vi "App - analyze RUS V6.vi"() -> ()   [LabVIEW 2021] (continued)
{"temperature"=59.124, "temperature str"="59.12400", "file path"=path "D:/Data/Ultrasound/LSCO/LSCO22__130814c/5_Cooling_2nd_try/September_2014/091714/59.12400K_500_2500_2.10000V_0.00000T_Sep17-2014__08-44-26_001_091714.bin", "last mod"=timestamp(3493802666 s since 1904-01-01), "file name str"="D:\\Data\\Ultrasound\\LSCO\\LSCO22__130814c\\5_Cooling_2nd_try\\September_2014\\091714\\59.12400K_500_2500_2.10000V_0.00000T_Sep17-2014__08-44-26_001_091714.bin", "mod time(min)"=58230044.43333333, "file format"=enum."binary", "power(V)"=2.1, "Magn Field(T) "=0.0}, {"temperature"=59.067, "temperature str"="59.06700", "file path"=path "D:/Data/Ultrasound/LSCO/LSCO22__130814c/5_Cooling_2nd_try/September_2014/091714/59.06700K_500_2500_2.10000V_0.00000T_Sep17-2014__08-45-45_001_091714.bin", "last mod"=timestamp(3493802745 s since 1904-01-01), "file name str"="D:\\Data\\Ultrasound\\LSCO\\LSCO22__130814c\\5_Cooling_2nd_try\\September_2014\\091714\\59.06700K_500_2500_2.10000V_0.00000T_Sep17-2014__08-45-45_001_091714.bin", "mod time(min)"=58230045.75, "file format"=enum."binary", "power(V)"=2.1, "Magn Field(T) "=0.0}, {"temperature"=59.005, "temperature str"="59.00500", "file path"=path "D:/Data/Ultrasound/LSCO/LSCO22__130814c/5_Cooling_2nd_try/September_2014/091714/59.00500K_500_2500_2.10000V_0.00000T_Sep17-2014__08-47-05_001_091714.bin", "last mod"=timestamp(3493802825 s since 1904-01-01), "file name str"="D:\\Data\\Ultrasound\\LSCO\\LSCO22__130814c\\5_Cooling_2nd_try\\September_2014\\091714\\59.00500K_500_2500_2.10000V_0.00000T_Sep17-2014__08-47-05_001_091714.bin", "mod time(min)"=58230047.083333336, "file format"=enum."binary", "power(V)"=2.1, "Magn Field(T) "=0.0}, {"temperature"=58.947, "temperature str"="58.94700", "file path"=path "D:/Data/Ultrasound/LSCO/LSCO22__130814c/5_Cooling_2nd_try/September_2014/091714/58.94700K_500_2500_2.10000V_0.00000T_Sep17-2014__08-48-24_001_091714.bin", "last mod"=timestamp(3493802904 s since 1904-01-01), "file name str"="D:\\Data\\Ultrasound\\LSCO\\LSCO22__130814c\\5_Cooling_2nd_try\\September_2014\\091714\\58.94700K_500_2500_2.10000V_0.00000T_Sep17-2014__08-48-24_001_091714.bin", "mod time(min)"=58230048.4, "file format"=enum."binary", "power(V)"=2.1, "Magn Field(T) "=0.0}, {"temperature"=58.886, "temperature str"="58.88600", "file path"=path "D:/Data/Ultrasound/LSCO/LSCO22__130814c/5_Cooling_2nd_try/September_2014/091714/58.88600K_500_2500_2.10000V_0.00000T_Sep17-2014__08-49-43_001_091714.bin", "last mod"=timestamp(3493802983 s since 1904-01-01), "file name str"="D:\\Data\\Ultrasound\\LSCO\\LSCO22__130814c\\5_Cooling_2nd_try\\September_2014\\091714\\58.88600K_500_2500_2.10000V_0.00000T_Sep17-2014__08-49-43_001_091714.bin", "mod time(min)"=58230049.71666667, "file format"=enum."binary", "power(V)"=2.1, "Magn Field(T) "=0.0}, {"temperature"=58.831, "temperature str"="58.83100", "file path"=path "D:/Data/Ultrasound/LSCO/LSCO22__130814c/5_Cooling_2nd_try/September_2014/091714/58.83100K_500_2500_2.10000V_0.00000T_Sep17-2014__08-51-03_001_091714.bin", "last mod"=timestamp(3493803063 s since 1904-01-01), "file name str"="D:\\Data\\Ultrasound\\LSCO\\LSCO22__130814c\\5_Cooling_2nd_try\\September_2014\\091714\\58.83100K_500_2500_2.10000V_0.00000T_Sep17-2014__08-51-03_001_091714.bin", "mod time(min)"=58230051.05, "file format"=enum."binary", "power(V)"=2.1, "Magn Field(T) "=0.0}, {"temperature"=58.769, "temperature str"="58.76900", "file path"=path "D:/Data/Ultrasound/LSCO/LSCO22__130814c/5_Cooling_2nd_try/September_2014/091714/58.76900K_500_2500_2.10000V_0.00000T_Sep17-2014__08-52-22_001_091714.bin", "last mod"=timestamp(3493803142 s since 1904-01-01), "file name str"="D:\\Data\\Ultrasound\\LSCO\\LSCO22__130814c\\5_Cooling_2nd_try\\September_2014\\091714\\58.76900K_500_2500_2.10000V_0.00000T_Sep17-2014__08-52-22_001_091714.bin", "mod time(min)"=58230052.36666667, "file format"=enum."binary", "power(V)"=2.1, "Magn Field(T) "=0.0}, {"temperature"=58.708, "temperature str"="58.70800", "file path"=path "D:/Data/Ultrasound/LSCO/LSCO22__130814c/5_Cooling_2nd_try/September_2014/091714/58.70800K_500_2500_2.10000V_0.00000T_Sep17-2014__08-53-41_001_091714.bin", "last mod"=timestamp(3493803221 s since 1904-01-01), "file name str"="D:\\Data\\Ultrasound\\LSCO\\LSCO22__130814c\\5_Cooling_2nd_try\\September_2014\\091714\\58.70800K_500_2500_2.10000V_0.00000T_Sep17-2014__08-53-41_001_091714.bin", "mod time(min)"=58230053.68333333, "file format"=enum."binary", "power(V)"=2.1, "Magn Field(T) "=0.0}, {"temperature"=58.65, "temperature str"="58.65000", "file path"=path "D:/Data/Ultrasound/LSCO/LSCO22__130814c/5_Cooling_2nd_try/September_2014/091714/58.65000K_500_2500_2.10000V_0.00000T_Sep17-2014__08-55-01_001_091714.bin", "last mod"=timestamp(3493803301 s since 1904-01-01), "file name str"="D:\\Data\\Ultrasound\\LSCO\\LSCO22__130814c\\5_Cooling_2nd_try\\September_2014\\091714\\58.65000K_500_2500_2.10000V_0.00000T_Sep17-2014__08-55-01_001_091714.bin", "mod time(min)"=58230055.016666666, "file format"=enum."binary", "power(V)"=2.1, "Magn Field(T) "=0.0}, {"temperature"=58.59, "temperature str"="58.59000", "file path"=path "D:/Data/Ultrasound/LSCO/LSCO22__130814c/5_Cooling_2nd_try/September_2014/091714/58.59000K_500_2500_2.10000V_0.00000T_Sep17-2014__08-56-20_001_091714.bin", "last mod"=timestamp(3493803380 s since 1904-01-01), "file name str"="D:\\Data\\Ultrasound\\LSCO\\LSCO22__130814c\\5_Cooling_2nd_try\\September_2014\\091714\\58.59000K_500_2500_2.10000V_0.00000T_Sep17-2014__08-56-20_001_091714.bin", "mod time(min)"=58230056.333333336, "file format"=enum."binary", "power(V)"=2.1, "Magn Field(T) "=0.0}, {"temperature"=58.53, "temperature str"="58.53000", "file path"=path "D:/Data/Ultrasound/LSCO/LSCO22__130814c/5_Cooling_2nd_try/September_2014/091714/58.53000K_500_2500_2.10000V_0.00000T_Sep17-2014__08-57-40_001_091714.bin", "last mod"=timestamp(3493803460 s since 1904-01-01), "file name str"="D:\\Data\\Ultrasound\\LSCO\\LSCO22__130814c\\5_Cooling_2nd_try\\September_2014\\091714\\58.53000K_500_2500_2.10000V_0.00000T_Sep17-2014__08-57-40_001_091714.bin", "mod time(min)"=58230057.666666664, "file format"=enum."binary", "power(V)"=2.1, "Magn Field(T) "=0.0}, {"temperature"=58.469, "temperature str"="58.46900", "file path"=path "D:/Data/Ultrasound/LSCO/LSCO22__130814c/5_Cooling_2nd_try/September_2014/091714/58.46900K_500_2500_2.10000V_0.00000T_Sep17-2014__08-58-59_001_091714.bin", "last mod"=timestamp(3493803539 s since 1904-01-01), "file name str"="D:\\Data\\Ultrasound\\LSCO\\LSCO22__130814c\\5_Cooling_2nd_try\\September_2014\\091714\\58.46900K_500_2500_2.10000V_0.00000T_Sep17-2014__08-58-59_001_091714.bin", "mod time(min)"=58230058.983333334, "file format"=enum."binary", "power(V)"=2.1, "Magn Field(T) "=0.0}, {"temperature"=58.41, "temperature str"="58.41000", "file path"=path "D:/Data/Ultrasound/LSCO/LSCO22__130814c/5_Cooling_2nd_try/September_2014/091714/58.41000K_500_2500_2.10000V_0.00000T_Sep17-2014__09-00-18_001_091714.bin", "last mod"=timestamp(3493803618 s since 1904-01-01), "file name str"="D:\\Data\\Ultrasound\\LSCO\\LSCO22__130814c\\5_Cooling_2nd_try\\September_2014\\091714\\58.41000K_500_2500_2.10000V_0.00000T_Sep17-2014__09-00-18_001_091714.bin", "mod time(min)"=58230060.3, "file format"=enum."binary", "power(V)"=2.1, "Magn Field(T) "=0.0}, {"temperature"=58.353, "temperature str"="58.35300", "file path"=path "D:/Data/Ultrasound/LSCO/LSCO22__130814c/5_Cooling_2nd_try/September_2014/091714/58.35300K_500_2500_2.10000V_0.00000T_Sep17-2014__09-01-38_001_091714.bin", "last mod"=timestamp(3493803698 s since 1904-01-01), "file name str"="D:\\Data\\Ultrasound\\LSCO\\LSCO22__130814c\\5_Cooling_2nd_try\\September_2014\\091714\\58.35300K_500_2500_2.10000V_0.00000T_Sep17-2014__09-01-38_001_091714.bin", "mod time(min)"=58230061.63333333, "file format"=enum."binary", "power(V)"=2.1, "Magn Field(T) "=0.0}, {"temperature"=58.289, "temperature str"="58.28900", "file path"=path "D:/Data/Ultrasound/LSCO/LSCO22__130814c/5_Cooling_2nd_try/September_2014/091714/58.28900K_500_2500_2.10000V_0.00000T_Sep17-2014__09-02-57_001_091714.bin", "last mod"=timestamp(3493803777 s since 1904-01-01), "file name str"="D:\\Data\\Ultrasound\\LSCO\\LSCO22__130814c\\5_Cooling_2nd_try\\September_2014\\091714\\58.28900K_500_2500_2.10000V_0.00000T_Sep17-2014__09-02-57_001_091714.bin", "mod time(min)"=58230062.95, "file format"=enum."binary", "power(V)"=2.1, "Magn Field(T) "=0.0}, {"temperature"=58.232, "temperature str"="58.23200", "file path"=path "D:/Data/Ultrasound/LSCO/LSCO22__130814c/5_Cooling_2nd_try/September_2014/091714/58.23200K_500_2500_2.10000V_0.00000T_Sep17-2014__09-04-17_001_091714.bin", "last mod"=timestamp(3493803857 s since 1904-01-01), "file name str"="D:\\Data\\Ultrasound\\LSCO\\LSCO22__130814c\\5_Cooling_2nd_try\\September_2014\\091714\\58.23200K_500_2500_2.10000V_0.00000T_Sep17-2014__09-04-17_001_091714.bin", "mod time(min)"=58230064.28333333, "file format"=enum."binary", "power(V)"=2.1, "Magn Field(T) "=0.0}, {"temperature"=58.173, "temperature str"="58.17300", "file path"=path "D:/Data/Ultrasound/LSCO/LSCO22__130814c/5_Cooling_2nd_try/September_2014/091714/58.17300K_500_2500_2.10000V_0.00000T_Sep17-2014__09-05-36_001_091714.bin", "last mod"=timestamp(3493803936 s since 1904-01-01), "file name str"="D:\\Data\\Ultrasound\\LSCO\\LSCO22__130814c\\5_Cooling_2nd_try\\September_2014\\091714\\58.17300K_500_2500_2.10000V_0.00000T_Sep17-2014__09-05-36_001_091714.bin", "mod time(min)"=58230065.6, "file format"=enum."binary", "power(V)"=2.1, "Magn Field(T) "=0.0}, {"temperature"=58.111, "temperature str"="58.11100", "file path"=path "D:/Data/Ultrasound/LSCO/LSCO22__130814c/5_Cooling_2nd_try/September_2014/091714/58.11100K_500_2500_2.10000V_0.00000T_Sep17-2014__09-06-55_001_091714.bin", "last mod"=timestamp(3493804015 s since 1904-01-01), "file name str"="D:\\Data\\Ultrasound\\LSCO\\LSCO22__130814c\\5_Cooling_2nd_try\\September_2014\\091714\\58.11100K_500_2500_2.10000V_0.00000T_Sep17-2014__09-06-55_001_091714.bin", "mod time(min)"=58230066.916666664, "file format"=enum."binary", "power(V)"=2.1, "Magn Field(T) "=0.0}, {"temperature"=58.052, "temperature str"="58.05200", "file path"=path "D:/Data/Ultrasound/LSCO/LSCO22__130814c/5_Cooling_2nd_try/September_2014/091714/58.05200K_500_2500_2.10000V_0.00000T_Sep17-2014__09-08-15_001_091714.bin", "last mod"=timestamp(3493804095 s since 1904-01-01), "file name str"="D:\\Data\\Ultrasound\\LSCO\\LSCO22__130814c\\5_Cooling_2nd_try\\September_2014\\091714\\58.05200K_500_2500_2.10000V_0.00000T_Sep17-2014__09-08-15_001_091714.bin", "mod time(min)"=58230068.25, "file format"=enum."binary", "power(V)"=2.1, "Magn Field(T) "=0.0}, {"temperature"=57.991, "temperature str"="57.99100", "file path"=path "D:/Data/Ultrasound/LSCO/LSCO22__130814c/5_Cooling_2nd_try/September_2014/091714/57.99100K_500_2500_2.10000V_0.00000T_Sep17-2014__09-09-34_001_091714.bin", "last mod"=timestamp(3493804174 s since 1904-01-01), "file name str"="D:\\Data\\Ultrasound\\LSCO\\LSCO22__130814c\\5_Cooling_2nd_try\\September_2014\\091714\\57.99100K_500_2500_2.10000V_0.00000T_Sep17-2014__09-09-34_001_091714.bin", "mod time(min)"=58230069.56666667, "file format"=enum."binary", "power(V)"=2.1, "Magn Field(T) "=0.0}, {"temperature"=57.933, "temperature str"="57.93300", "file path"=path "D:/Data/Ultrasound/LSCO/LSCO22__130814c/5_Cooling_2nd_try/September_2014/091714/57.93300K_500_2500_2.10000V_0.00000T_Sep17-2014__09-10-53_001_091714.bin", "last mod"=timestamp(3493804253 s since 1904-01-01), "file name str"="D:\\Data\\Ultrasound\\LSCO\\LSCO22__130814c\\5_Cooling_2nd_try\\September_2014\\091714\\57.93300K_500_2500_2.10000V_0.00000T_Sep17-2014__09-10-53_001_091714.bin", "mod time(min)"=58230070.88333333, "file format"=enum."binary", "power(V)"=2.1, "Magn Field(T) "=0.0}, {"temperature"=57.871, "temperature str"="57.87100", "file path"=path "D:/Data/Ultrasound/LSCO/LSCO22__130814c/5_Cooling_2nd_try/September_2014/091714/57.87100K_500_2500_2.10000V_0.00000T_Sep17-2014__09-12-13_001_091714.bin", "last mod"=timestamp(3493804333 s since 1904-01-01), "file name str"="D:\\Data\\Ultrasound\\LSCO\\LSCO22__130814c\\5_Cooling_2nd_try\\September_2014\\091714\\57.87100K_500_2500_2.10000V_0.00000T_Sep17-2014__09-12-13_001_091714.bin", "mod time(min)"=58230072.21666667, "file format"=enum."binary", "power(V)"=2.1, "Magn Field(T) "=0.0}, {"temperature"=57.811, "temperature str"="57.81100", "file path"=path "D:/Data/Ultrasound/LSCO/LSCO22__130814c/5_Cooling_2nd_try/September_2014/091714/57.81100K_500_2500_2.10000V_0.00000T_Sep17-2014__09-13-32_001_091714.bin", "last mod"=timestamp(3493804412 s since 1904-01-01), "file name str"="D:\\Data\\Ultrasound\\LSCO\\LSCO22__130814c\\5_Cooling_2nd_try\\September_2014\\091714\\57.81100K_500_2500_2.10000V_0.00000T_Sep17-2014__09-13-32_001_091714.bin", "mod time(min)"=58230073.53333333, "file format"=enum."binary", "power(V)"=2.1, "Magn Field(T) "=0.0}, {"temperature"=57.752, "temperature str"="57.75200", "file path"=path "D:/Data/Ultrasound/LSCO/LSCO22__130814c/5_Cooling_2nd_try/September_2014/091714/57.75200K_500_2500_2.10000V_0.00000T_Sep17-2014__09-14-52_001_091714.bin", "last mod"=timestamp(3493804492 s since 1904-01-01), "file name str"="D:\\Data\\Ultrasound\\LSCO\\LSCO22__130814c\\5_Cooling_2nd_try\\September_2014\\091714\\57.75200K_500_2500_2.10000V_0.00000T_Sep17-2014__09-14-52_001_091714.bin", "mod time(min)"=58230074.86666667, "file format"=enum."binary", "power(V)"=2.1, "Magn Field(T) "=0.0}, {"temperature"=57.689, "temperature str"="57.68900", "file path"=path "D:/Data/Ultrasound/LSCO/LSCO22__130814c/5_Cooling_2nd_try/September_2014/091714/57.68900K_500_2500_2.10000V_0.00000T_Sep17-2014__09-16-11_001_091714.bin", "last mod"=timestamp(3493804571 s since 1904-01-01), "file name str"="D:\\Data\\Ultrasound\\LSCO\\LSCO22__130814c\\5_Cooling_2nd_try\\September_2014\\091714\\57.68900K_500_2500_2.10000V_0.00000T_Sep17-2014__09-16-11_001_091714.bin", "mod time(min)"=58230076.18333333, "file format"=enum."binary", "power(V)"=2.1, "Magn Field(T) "=0.0}, {"temperature"=57.629, "temperature str"="57.62900", "file path"=path "D:/Data/Ultrasound/LSCO/LSCO22__130814c/5_Cooling_2nd_try/September_2014/091714/57.62900K_500_2500_2.10000V_0.00000T_Sep17-2014__09-17-30_001_091714.bin", "last mod"=timestamp(3493804650 s since 1904-01-01), "file name str"="D:\\Data\\Ultrasound\\LSCO\\LSCO22__130814c\\5_Cooling_2nd_try\\September_2014\\091714\\57.62900K_500_2500_2.10000V_0.00000T_Sep17-2014__09-17-30_001_091714.bin", "mod time(min)"=58230077.5, "file format"=enum."binary", "power(V)"=2.1, "Magn Field(T) "=0.0}, {"temperature"=57.57, "temperature str"="57.57000", "file path"=path "D:/Data/Ultrasound/LSCO/LSCO22__130814c/5_Cooling_2nd_try/September_2014/091714/57.57000K_500_2500_2.10000V_0.00000T_Sep17-2014__09-18-50_001_091714.bin", "last mod"=timestamp(3493804730 s since 1904-01-01), "file name str"="D:\\Data\\Ultrasound\\LSCO\\LSCO22__130814c\\5_Cooling_2nd_try\\September_2014\\091714\\57.57000K_500_2500_2.10000V_0.00000T_Sep17-2014__09-18-50_001_091714.bin", "mod time(min)"=58230078.833333336, "file format"=enum."binary", "power(V)"=2.1, "Magn Field(T) "=0.0}, {"temperature"=57.51, "temperature str"="57.51000", "file path"=path "D:/Data/Ultrasound/LSCO/LSCO22__130814c/5_Cooling_2nd_try/September_2014/091714/57.51000K_500_2500_2.10000V_0.00000T_Sep17-2014__09-20-09_001_091714.bin", "last mod"=timestamp(3493804809 s since 1904-01-01), "file name str"="D:\\Data\\Ultrasound\\LSCO\\LSCO22__130814c\\5_Cooling_2nd_try\\September_2014\\091714\\57.51000K_500_2500_2.10000V_0.00000T_Sep17-2014__09-20-09_001_091714.bin", "mod time(min)"=58230080.15, "file format"=enum."binary", "power(V)"=2.1, "Magn Field(T) "=0.0}, {"temperature"=57.452, "temperature str"="57.45200", "file path"=path "D:/Data/Ultrasound/LSCO/LSCO22__130814c/5_Cooling_2nd_try/September_2014/091714/57.45200K_500_2500_2.10000V_0.00000T_Sep17-2014__09-21-28_001_091714.bin", "last mod"=timestamp(3493804888 s since 1904-01-01), "file name str"="D:\\Data\\Ultrasound\\LSCO\\LSCO22__130814c\\5_Cooling_2nd_try\\September_2014\\091714\\57.45200K_500_2500_2.10000V_0.00000T_Sep17-2014__09-21-28_001_091714.bin", "mod time(min)"=58230081.46666667, "file format"=enum."binary", "power(V)"=2.1, "Magn Field(T) "=0.0}, {"temperature"=57.391, "temperature str"="57.39100", "file path"=path "D:/Data/Ultrasound/LSCO/LSCO22__130814c/5_Cooling_2nd_try/September_2014/091714/57.39100K_500_2500_2.10000V_0.00000T_Sep17-2014__09-22-48_001_091714.bin", "last mod"=timestamp(3493804968 s since 1904-01-01), "file name str"="D:\\Data\\Ultrasound\\LSCO\\LSCO22__130814c\\5_Cooling_2nd_try\\September_2014\\091714\\57.39100K_500_2500_2.10000V_0.00000T_Sep17-2014__09-22-48_001_091714.bin", "mod time(min)"=58230082.8, "file format"=enum."binary", "power(V)"=2.1, "Magn Field(T) "=0.0}, {"temperature"=57.328, "temperature str"="57.32800", "file path"=path "D:/Data/Ultrasound/LSCO/LSCO22__130814c/5_Cooling_2nd_try/September_2014/091714/57.32800K_500_2500_2.10000V_0.00000T_Sep17-2014__09-24-07_001_091714.bin", "last mod"=timestamp(3493805047 s since 1904-01-01), "file name str"="D:\\Data\\Ultrasound\\LSCO\\LSCO22__130814c\\5_Cooling_2nd_try\\September_2014\\091714\\57.32800K_500_2500_2.10000V_0.00000T_Sep17-2014__09-24-07_001_091714.bin", "mod time(min)"=58230084.11666667, "file format"=enum."binary", "power(V)"=2.1, "Magn Field(T) "=0.0}, {"temperature"=57.27, "temperature str"="57.27000", "file path"=path "D:/Data/Ultrasound/LSCO/LSCO22__130814c/5_Cooling_2nd_try/September_2014/091714/57.27000K_500_2500_2.10000V_0.00000T_Sep17-2014__09-25-27_001_091714.bin", "last mod"=timestamp(3493805127 s since 1904-01-01), "file name str"="D:\\Data\\Ultrasound\\LSCO\\LSCO22__130814c\\5_Cooling_2nd_try\\September_2014\\091714\\57.27000K_500_2500_2.10000V_0.00000T_Sep17-2014__09-25-27_001_091714.bin", "mod time(min)"=58230085.45, "file format"=enum."binary", "power(V)"=2.1, "Magn Field(T) "=0.0}, {"temperature"=57.209, "temperature str"="57.20900", "file path"=path "D:/Data/Ultrasound/LSCO/LSCO22__130814c/5_Cooling_2nd_try/September_2014/091714/57.20900K_500_2500_2.10000V_0.00000T_Sep17-2014__09-26-46_001_091714.bin", "last mod"=timestamp(3493805206 s since 1904-01-01), "file name str"="D:\\Data\\Ultrasound\\LSCO\\LSCO22__130814c\\5_Cooling_2nd_try\\September_2014\\091714\\57.20900K_500_2500_2.10000V_0.00000T_Sep17-2014__09-26-46_001_091714.bin", "mod time(min)"=58230086.766666666, "file format"=enum."binary", "power(V)"=2.1, "Magn Field(T) "=0.0}, {"temperature"=57.149, "temperature str"="57.14900", "file path"=path "D:/Data/Ultrasound/LSCO/LSCO22__130814c/5_Cooling_2nd_try/September_2014/091714/57.14900K_500_2500_2.10000V_0.00000T_Sep17-2014__09-28-05_001_091714.bin", "last mod"=timestamp(3493805285 s since 1904-01-01), "file name str"="D:\\Data\\Ultrasound\\LSCO\\LSCO22__130814c\\5_Cooling_2nd_try\\September_2014\\091714\\57.14900K_500_2500_2.10000V_0.00000T_Sep17-2014__09-28-05_001_091714.bin", "mod time(min)"=58230088.083333336, "file format"=enum."binary", "power(V)"=2.1, "Magn Field(T) "=0.0}, {"temperature"=57.087, "temperature str"="57.08700", "file path"=path "D:/Data/Ultrasound/LSCO/LSCO22__130814c/5_Cooling_2nd_try/September_2014/091714/57.08700K_500_2500_2.10000V_0.00000T_Sep17-2014__09-29-25_001_091714.bin", "last mod"=timestamp(3493805365 s since 1904-01-01), "file name str"="D:\\Data\\Ultrasound\\LSCO\\LSCO22__130814c\\5_Cooling_2nd_try\\September_2014\\091714\\57.08700K_500_2500_2.10000V_0.00000T_Sep17-2014__09-29-25_001_091714.bin", "mod time(min)"=58230089.416666664, "file format"=enum."binary", "power(V)"=2.1, "Magn Field(T) "=0.0}, {"temperature"=57.027, "temperature str"="57.02700", "file path"=path "D:/Data/Ultrasound/LSCO/LSCO22__130814c/5_Cooling_2nd_try/September_2014/091714/57.02700K_500_2500_2.10000V_0.00000T_Sep17-2014__09-30-44_001_091714.bin", "last mod"=timestamp(3493805444 s since 1904-01-01), "file name str"="D:\\Data\\Ultrasound\\LSCO\\LSCO22__130814c\\5_Cooling_2nd_try\\September_2014\\091714\\57.02700K_500_2500_2.10000V_0.00000T_Sep17-2014__09-30-44_001_091714.bin", "mod time(min)"=58230090.733333334, "file format"=enum."binary", "power(V)"=2.1, "Magn Field(T) "=0.0}, {"temperature"=56.968, "temperature str"="56.96800", "file path"=path "D:/Data/Ultrasound/LSCO/LSCO22__130814c/5_Cooling_2nd_try/September_2014/091714/56.96800K_500_2500_2.10000V_0.00000T_Sep17-2014__09-32-04_001_091714.bin", "last mod"=timestamp(3493805524 s since 1904-01-01), "file name str"="D:\\Data\\Ultrasound\\LSCO\\LSCO22__130814c\\5_Cooling_2nd_try\\September_2014\\091714\\56.96800K_500_2500_2.10000V_0.00000T_Sep17-2014__09-32-04_001_091714.bin", "mod time(min)"=58230092.06666667, "file format"=enum."binary", "power(V)"=2.1, "Magn Field(T) "=0.0}, {"temperature"=56.903, "temperature str"="56.90300", "file path"=path "D:/Data/Ultrasound/LSCO/LSCO22__130814c/5_Cooling_2nd_try/September_2014/091714/56.90300K_500_2500_2.10000V_0.00000T_Sep17-2014__09-33-23_001_091714.bin", "last mod"=timestamp(3493805603 s since 1904-01-01), "file name str"="D:\\Data\\Ultrasound\\LSCO\\LSCO22__130814c\\5_Cooling_2nd_try\\September_2014\\091714\\56.90300K_500_2500_2.10000V_0.00000T_Sep17-2014__09-33-23_001_091714.bin", "mod time(min)"=58230093.38333333, "file format"=enum."binary", "power(V)"=2.1, "Magn Field(T) "=0.0}, {"temperature"=56.847, "temperature str"="56.84700", "file path"=path "D:/Data/Ultrasound/LSCO/LSCO22__130814c/5_Cooling_2nd_try/September_2014/091714/56.84700K_500_2500_2.10000V_0.00000T_Sep17-2014__09-34-42_001_091714.bin", "last mod"=timestamp(3493805682 s since 1904-01-01), "file name str"="D:\\Data\\Ultrasound\\LSCO\\LSCO22__130814c\\5_Cooling_2nd_try\\September_2014\\091714\\56.84700K_500_2500_2.10000V_0.00000T_Sep17-2014__09-34-42_001_091714.bin", "mod time(min)"=58230094.7, "file format"=enum."binary", "power(V)"=2.1, "Magn Field(T) "=0.0}, {"temperature"=56.789, "temperature str"="56.78900", "file path"=path "D:/Data/Ultrasound/LSCO/LSCO22__130814c/5_Cooling_2nd_try/September_2014/091714/56.78900K_500_2500_2.10000V_0.00000T_Sep17-2014__09-36-02_001_091714.bin", "last mod"=timestamp(3493805762 s since 1904-01-01), "file name str"="D:\\Data\\Ultrasound\\LSCO\\LSCO22__130814c\\5_Cooling_2nd_try\\September_2014\\091714\\56.78900K_500_2500_2.10000V_0.00000T_Sep17-2014__09-36-02_001_091714.bin", "mod time(min)"=58230096.03333333, "file format"=enum."binary", "power(V)"=2.1, "Magn Field(T) "=0.0}, {"temperature"=56.72, "temperature str"="56.72000", "file path"=path "D:/Data/Ultrasound/LSCO/LSCO22__130814c/5_Cooling_2nd_try/September_2014/091714/56.72000K_500_2500_2.10000V_0.00000T_Sep17-2014__09-37-21_001_091714.bin", "last mod"=timestamp(3493805841 s since 1904-01-01), "file name str"="D:\\Data\\Ultrasound\\LSCO\\LSCO22__130814c\\5_Cooling_2nd_try\\September_2014\\091714\\56.72000K_500_2500_2.10000V_0.00000T_Sep17-2014__09-37-21_001_091714.bin", "mod time(min)"=58230097.35, "file format"=enum."binary", "power(V)"=2.1, "Magn Field(T) "=0.0}, {"temperature"=56.664, "temperature str"="56.66400", "file path"=path "D:/Data/Ultrasound/LSCO/LSCO22__130814c/5_Cooling_2nd_try/September_2014/091714/56.66400K_500_2500_2.10000V_0.00000T_Sep17-2014__09-38-40_001_091714.bin", "last mod"=timestamp(3493805920 s since 1904-01-01), "file name str"="D:\\Data\\Ultrasound\\LSCO\\LSCO22__130814c\\5_Cooling_2nd_try\\September_2014\\091714\\56.66400K_500_2500_2.10000V_0.00000T_Sep17-2014__09-38-40_001_091714.bin", "mod time(min)"=58230098.666666664, "file format"=enum."binary", "power(V)"=2.1, "Magn Field(T) "=0.0}, {"temperature"=56.602, "temperature str"="56.60200", "file path"=path "D:/Data/Ultrasound/LSCO/LSCO22__130814c/5_Cooling_2nd_try/September_2014/091714/56.60200K_500_2500_2.10000V_0.00000T_Sep17-2014__09-40-00_001_091714.bin", "last mod"=timestamp(3493806000 s since 1904-01-01), "file name str"="D:\\Data\\Ultrasound\\LSCO\\LSCO22__130814c\\5_Cooling_2nd_try\\September_2014\\091714\\56.60200K_500_2500_2.10000V_0.00000T_Sep17-2014__09-40-00_001_091714.bin", "mod time(min)"=58230100.0, "file format"=enum."binary", "power(V)"=2.1, "Magn Field(T) "=0.0}, {"temperature"=56.543, "temperature str"="56.54300", "file path"=path "D:/Data/Ultrasound/LSCO/LSCO22__130814c/5_Cooling_2nd_try/September_2014/091714/56.54300K_500_2500_2.10000V_0.00000T_Sep17-2014__09-41-19_001_091714.bin", "last mod"=timestamp(3493806079 s since 1904-01-01), "file name str"="D:\\Data\\Ultrasound\\LSCO\\LSCO22__130814c\\5_Cooling_2nd_try\\September_2014\\091714\\56.54300K_500_2500_2.10000V_0.00000T_Sep17-2014__09-41-19_001_091714.bin", "mod time(min)"=58230101.31666667, "file format"=enum."binary", "power(V)"=2.1, "Magn Field(T) "=0.0}, {"temperature"=56.48, "temperature str"="56.48000", "file path"=path "D:/Data/Ultrasound/LSCO/LSCO22__130814c/5_Cooling_2nd_try/September_2014/091714/56.48000K_500_2500_2.10000V_0.00000T_Sep17-2014__09-42-39_001_091714.bin", "last mod"=timestamp(3493806159 s since 1904-01-01), "file name str"="D:\\Data\\Ultrasound\\LSCO\\LSCO22__130814c\\5_Cooling_2nd_try\\September_2014\\091714\\56.48000K_500_2500_2.10000V_0.00000T_Sep17-2014__09-42-39_001_091714.bin", "mod time(min)"=58230102.65, "file format"=enum."binary", "power(V)"=2.1, "Magn Field(T) "=0.0}, {"temperature"=56.419, "temperature str"="56.41900", "file path"=path "D:/Data/Ultrasound/LSCO/LSCO22__130814c/5_Cooling_2nd_try/September_2014/091714/56.41900K_500_2500_2.10000V_0.00000T_Sep17-2014__09-43-58_001_091714.bin", "last mod"=timestamp(3493806238 s since 1904-01-01), "file name str"="D:\\Data\\Ultrasound\\LSCO\\LSCO22__130814c\\5_Cooling_2nd_try\\September_2014\\091714\\56.41900K_500_2500_2.10000V_0.00000T_Sep17-2014__09-43-58_001_091714.bin", "mod time(min)"=58230103.96666667, "file format"=enum."binary", "power(V)"=2.1, "Magn Field(T) "=0.0}, {"temperature"=56.359, "temperature str"="56.35900", "file path"=path "D:/Data/Ultrasound/LSCO/LSCO22__130814c/5_Cooling_2nd_try/September_2014/091714/56.35900K_500_2500_2.10000V_0.00000T_Sep17-2014__09-45-17_001_091714.bin", "last mod"=timestamp(3493806317 s since 1904-01-01), "file name str"="D:\\Data\\Ultrasound\\LSCO\\LSCO22__130814c\\5_Cooling_2nd_try\\September_2014\\091714\\56.35900K_500_2500_2.10000V_0.00000T_Sep17-2014__09-45-17_001_091714.bin", "mod time(min)"=58230105.28333333, "file format"=enum."binary", "power(V)"=2.1, "Magn Field(T) "=0.0}, {"temperature"=56.297, "temperature str"="56.29700", "file path"=path "D:/Data/Ultrasound/LSCO/LSCO22__130814c/5_Cooling_2nd_try/September_2014/091714/56.29700K_500_2500_2.10000V_0.00000T_Sep17-2014__09-46-37_001_091714.bin", "last mod"=timestamp(3493806397 s since 1904-01-01), "file name str"="D:\\Data\\Ultrasound\\LSCO\\LSCO22__130814c\\5_Cooling_2nd_try\\September_2014\\091714\\56.29700K_500_2500_2.10000V_0.00000T_Sep17-2014__09-46-37_001_091714.bin", "mod time(min)"=58230106.61666667, "file format"=enum."binary", "power(V)"=2.1, "Magn Field(T) "=0.0}, {"temperature"=56.237, "temperature str"="56.23700", "file path"=path "D:/Data/Ultrasound/LSCO/LSCO22__130814c/5_Cooling_2nd_try/September_2014/091714/56.23700K_500_2500_2.10000V_0.00000T_Sep17-2014__09-47-56_001_091714.bin", "last mod"=timestamp(3493806476 s since 1904-01-01), "file name str"="D:\\Data\\Ultrasound\\LSCO\\LSCO22__130814c\\5_Cooling_2nd_try\\September_2014\\091714\\56.23700K_500_2500_2.10000V_0.00000T_Sep17-2014__09-47-56_001_091714.bin", "mod time(min)"=58230107.93333333, "file format"=enum."binary", "power(V)"=2.1, "Magn Field(T) "=0.0}, {"temperature"=56.174, "temperature str"="56.17400", "file path"=path "D:/Data/Ultrasound/LSCO/LSCO22__130814c/5_Cooling_2nd_try/September_2014/091714/56.17400K_500_2500_2.10000V_0.00000T_Sep17-2014__09-49-16_001_091714.bin", "last mod"=timestamp(3493806556 s since 1904-01-01), "file name str"="D:\\Data\\Ultrasound\\LSCO\\LSCO22__130814c\\5_Cooling_2nd_try\\September_2014\\091714\\56.17400K_500_2500_2.10000V_0.00000T_Sep17-2014__09-49-16_001_091714.bin", "mod time(min)"=58230109.266666666, "file format"=enum."binary", "power(V)"=2.1, "Magn Field(T) "=0.0}, {"temperature"=56.114, "temperature str"="56.11400", "file path"=path "D:/Data/Ultrasound/LSCO/LSCO22__130814c/5_Cooling_2nd_try/September_2014/091714/56.11400K_500_2500_2.10000V_0.00000T_Sep17-2014__09-50-35_001_091714.bin", "last mod"=timestamp(3493806635 s since 1904-01-01), "file name str"="D:\\Data\\Ultrasound\\LSCO\\LSCO22__130814c\\5_Cooling_2nd_try\\September_2014\\091714\\56.11400K_500_2500_2.10000V_0.00000T_Sep17-2014__09-50-35_001_091714.bin", "mod time(min)"=58230110.583333336, "file format"=enum."binary", "power(V)"=2.1, "Magn Field(T) "=0.0}, {"temperature"=56.051, "temperature str"="56.05100", "file path"=path "D:/Data/Ultrasound/LSCO/LSCO22__130814c/5_Cooling_2nd_try/September_2014/091714/56.05100K_500_2500_2.10000V_0.00000T_Sep17-2014__09-51-54_001_091714.bin", "last mod"=timestamp(3493806714 s since 1904-01-01), "file name str"="D:\\Data\\Ultrasound\\LSCO\\LSCO22__130814c\\5_Cooling_2nd_try\\September_2014\\091714\\56.05100K_500_2500_2.10000V_0.00000T_Sep17-2014__09-51-54_001_091714.bin", "mod time(min)"=58230111.9, "file format"=enum."binary", "power(V)"=2.1, "Magn Field(T) "=0.0}, {"temperature"=55.989, "temperature str"="55.98900", "file path"=path "D:/Data/Ultrasound/LSCO/LSCO22__130814c/5_Cooling_2nd_try/September_2014/091714/55.98900K_500_2500_2.10000V_0.00000T_Sep17-2014__09-53-14_001_091714.bin", "last mod"=timestamp(3493806794 s since 1904-01-01), "file name str"="D:\\Data\\Ultrasound\\LSCO\\LSCO22__130814c\\5_Cooling_2nd_try\\September_2014\\091714\\55.98900K_500_2500_2.10000V_0.00000T_Sep17-2014__09-53-14_001_091714.bin", "mod time(min)"=58230113.233333334, "file format"=enum."binary", "power(V)"=2.1, "Magn Field(T) "=0.0}, {"temperature"=55.93, "temperature str"="55.93000", "file path"=path "D:/Data/Ultrasound/LSCO/LSCO22__130814c/5_Cooling_2nd_try/September_2014/091714/55.93000K_500_2500_2.10000V_0.00000T_Sep17-2014__09-54-33_001_091714.bin", "last mod"=timestamp(3493806873 s since 1904-01-01), "file name str"="D:\\Data\\Ultrasound\\LSCO\\LSCO22__130814c\\5_Cooling_2nd_try\\September_2014\\091714\\55.93000K_500_2500_2.10000V_0.00000T_Sep17-2014__09-54-33_001_091714.bin", "mod time(min)"=58230114.55, "file format"=enum."binary", "power(V)"=2.1, "Magn Field(T) "=0.0}, {"temperature"=55.865, "temperature str"="55.86500", "file path"=path "D:/Data/Ultrasound/LSCO/LSCO22__130814c/5_Cooling_2nd_try/September_2014/091714/55.86500K_500_2500_2.10000V_0.00000T_Sep17-2014__09-55-52_001_091714.bin", "last mod"=timestamp(3493806952 s since 1904-01-01), "file name str"="D:\\Data\\Ultrasound\\LSCO\\LSCO22__130814c\\5_Cooling_2nd_try\\September_2014\\091714\\55.86500K_500_2500_2.10000V_0.00000T_Sep17-2014__09-55-52_001_091714.bin", "mod time(min)"=58230115.86666667, "file format"=enum."binary", "power(V)"=2.1, "Magn Field(T) "=0.0}, {"temperature"=55.805, "temperature str"="55.80500", "file path"=path "D:/Data/Ultrasound/LSCO/LSCO22__130814c/5_Cooling_2nd_try/September_2014/091714/55.80500K_500_2500_2.10000V_0.00000T_Sep17-2014__09-57-12_001_091714.bin", "last mod"=timestamp(3493807032 s since 1904-01-01), "file name str"="D:\\Data\\Ultrasound\\LSCO\\LSCO22__130814c\\5_Cooling_2nd_try\\September_2014\\091714\\55.80500K_500_2500_2.10000V_0.00000T_Sep17-2014__09-57-12_001_091714.bin", "mod time(min)"=58230117.2, "file format"=enum."binary", "power(V)"=2.1, "Magn Field(T) "=0.0}, {"temperature"=55.744, "temperature str"="55.74400", "file path"=path "D:/Data/Ultrasound/LSCO/LSCO22__130814c/5_Cooling_2nd_try/September_2014/091714/55.74400K_500_2500_2.10000V_0.00000T_Sep17-2014__09-58-31_001_091714.bin", "last mod"=timestamp(3493807111 s since 1904-01-01), "file name str"="D:\\Data\\Ultrasound\\LSCO\\LSCO22__130814c\\5_Cooling_2nd_try\\September_2014\\091714\\55.74400K_500_2500_2.10000V_0.00000T_Sep17-2014__09-58-31_001_091714.bin", "mod time(min)"=58230118.516666666, "file format"=enum."binary", "power(V)"=2.1, "Magn Field(T) "=0.0}, {"temperature"=55.681, "temperature str"="55.68100", "file path"=path "D:/Data/Ultrasound/LSCO/LSCO22__130814c/5_Cooling_2nd_try/September_2014/091714/55.68100K_500_2500_2.10000V_0.00000T_Sep17-2014__09-59-51_001_091714.bin", "last mod"=timestamp(3493807191 s since 1904-01-01), "file name str"="D:\\Data\\Ultrasound\\LSCO\\LSCO22__130814c\\5_Cooling_2nd_try\\September_2014\\091714\\55.68100K_500_2500_2.10000V_0.00000T_Sep17-2014__09-59-51_001_091714.bin", "mod time(min)"=58230119.85, "file format"=enum."binary", "power(V)"=2.1, "Magn Field(T) "=0.0}, {"temperature"=55.622, "temperature str"="55.62200", "file path"=path "D:/Data/Ultrasound/LSCO/LSCO22__130814c/5_Cooling_2nd_try/September_2014/091714/55.62200K_500_2500_2.10000V_0.00000T_Sep17-2014__10-01-10_001_091714.bin", "last mod"=timestamp(3493807270 s since 1904-01-01), "file name str"="D:\\Data\\Ultrasound\\LSCO\\LSCO22__130814c\\5_Cooling_2nd_try\\September_2014\\091714\\55.62200K_500_2500_2.10000V_0.00000T_Sep17-2014__10-01-10_001_091714.bin", "mod time(min)"=58230121.166666664, "file format"=enum."binary", "power(V)"=2.1, "Magn Field(T) "=0.0}, {"temperature"=55.56, "temperature str"="55.56000", "file path"=path "D:/Data/Ultrasound/LSCO/LSCO22__130814c/5_Cooling_2nd_try/September_2014/091714/55.56000K_500_2500_2.10000V_0.00000T_Sep17-2014__10-02-29_001_091714.bin", "last mod"=timestamp(3493807349 s since 1904-01-01), "file name str"="D:\\Data\\Ultrasound\\LSCO\\LSCO22__130814c\\5_Cooling_2nd_try\\September_2014\\091714\\55.56000K_500_2500_2.10000V_0.00000T_Sep17-2014__10-02-29_001_091714.bin", "mod time(min)"=58230122.483333334, "file format"=enum."binary", "power(V)"=2.1, "Magn Field(T) "=0.0}, {"temperature"=55.498, "temperature str"="55.49800", "file path"=path "D:/Data/Ultrasound/LSCO/LSCO22__130814c/5_Cooling_2nd_try/September_2014/091714/55.49800K_500_2500_2.10000V_0.00000T_Sep17-2014__10-03-49_001_091714.bin", "last mod"=timestamp(3493807429 s since 1904-01-01), "file name str"="D:\\Data\\Ultrasound\\LSCO\\LSCO22__130814c\\5_Cooling_2nd_try\\September_2014\\091714\\55.49800K_500_2500_2.10000V_0.00000T_Sep17-2014__10-03-49_001_091714.bin", "mod time(min)"=58230123.81666667, "file format"=enum."binary", "power(V)"=2.1, "Magn Field(T) "=0.0}, {"temperature"=55.437, "temperature str"="55.43700", "file path"=path "D:/Data/Ultrasound/LSCO/LSCO22__130814c/5_Cooling_2nd_try/September_2014/091714/55.43700K_500_2500_2.10000V_0.00000T_Sep17-2014__10-05-08_001_091714.bin", "last mod"=timestamp(3493807508 s since 1904-01-01), "file name str"="D:\\Data\\Ultrasound\\LSCO\\LSCO22__130814c\\5_Cooling_2nd_try\\September_2014\\091714\\55.43700K_500_2500_2.10000V_0.00000T_Sep17-2014__10-05-08_001_091714.bin", "mod time(min)"=58230125.13333333, "file format"=enum."binary", "power(V)"=2.1, "Magn Field(T) "=0.0}, {"temperature"=55.376, "temperature str"="55.37600", "file path"=path "D:/Data/Ultrasound/LSCO/LSCO22__130814c/5_Cooling_2nd_try/September_2014/091714/55.37600K_500_2500_2.10000V_0.00000T_Sep17-2014__10-06-27_001_091714.bin", "last mod"=timestamp(3493807587 s since 1904-01-01), "file name str"="D:\\Data\\Ultrasound\\LSCO\\LSCO22__130814c\\5_Cooling_2nd_try\\September_2014\\091714\\55.37600K_500_2500_2.10000V_0.00000T_Sep17-2014__10-06-27_001_091714.bin", "mod time(min)"=58230126.45, "file format"=enum."binary", "power(V)"=2.1, "Magn Field(T) "=0.0}, {"temperature"=55.311, "temperature str"="55.31100", "file path"=path "D:/Data/Ultrasound/LSCO/LSCO22__130814c/5_Cooling_2nd_try/September_2014/091714/55.31100K_500_2500_2.10000V_0.00000T_Sep17-2014__10-07-47_001_091714.bin", "last mod"=timestamp(3493807667 s since 1904-01-01), "file name str"="D:\\Data\\Ultrasound\\LSCO\\LSCO22__130814c\\5_Cooling_2nd_try\\September_2014\\091714\\55.31100K_500_2500_2.10000V_0.00000T_Sep17-2014__10-07-47_001_091714.bin", "mod time(min)"=58230127.78333333, "file format"=enum."binary", "power(V)"=2.1, "Magn Field(T) "=0.0}, {"temperature"=55.252, "temperature str"="55.25200", "file path"=path "D:/Data/Ultrasound/LSCO/LSCO22__130814c/5_Cooling_2nd_try/September_2014/091714/55.25200K_500_2500_2.10000V_0.00000T_Sep17-2014__10-09-06_001_091714.bin", "last mod"=timestamp(3493807746 s since 1904-01-01), "file name str"="D:\\Data\\Ultrasound\\LSCO\\LSCO22__130814c\\5_Cooling_2nd_try\\September_2014\\091714\\55.25200K_500_2500_2.10000V_0.00000T_Sep17-2014__10-09-06_001_091714.bin", "mod time(min)"=58230129.1, "file format"=enum."binary", "power(V)"=2.1, "Magn Field(T) "=0.0}, {"temperature"=55.188, "temperature str"="55.18800", "file path"=path "D:/Data/Ultrasound/LSCO/LSCO22__130814c/5_Cooling_2nd_try/September_2014/091714/55.18800K_500_2500_2.10000V_0.00000T_Sep17-2014__10-10-25_001_091714.bin", "last mod"=timestamp(3493807825 s since 1904-01-01), "file name str"="D:\\Data\\Ultrasound\\LSCO\\LSCO22__130814c\\5_Cooling_2nd_try\\September_2014\\091714\\55.18800K_500_2500_2.10000V_0.00000T_Sep17-2014__10-10-25_001_091714.bin", "mod time(min)"=58230130.416666664, "file format"=enum."binary", "power(V)"=2.1, "Magn Field(T) "=0.0}, {"temperature"=55.128, "temperature str"="55.12800", "file path"=path "D:/Data/Ultrasound/LSCO/LSCO22__130814c/5_Cooling_2nd_try/September_2014/091714/55.12800K_500_2500_2.10000V_0.00000T_Sep17-2014__10-11-45_001_091714.bin", "last mod"=timestamp(3493807905 s since 1904-01-01), "file name str"="D:\\Data\\Ultrasound\\LSCO\\LSCO22__130814c\\5_Cooling_2nd_try\\September_2014\\091714\\55.12800K_500_2500_2.10000V_0.00000T_Sep17-2014__10-11-45_001_091714.bin", "mod time(min)"=58230131.75, "file format"=enum."binary", "power(V)"=2.1, "Magn Field(T) "=0.0}, {"temperature"=55.063, "temperature str"="55.06300", "file path"=path "D:/Data/Ultrasound/LSCO/LSCO22__130814c/5_Cooling_2nd_try/September_2014/091714/55.06300K_500_2500_2.10000V_0.00000T_Sep17-2014__10-13-04_001_091714.bin", "last mod"=timestamp(3493807984 s since 1904-01-01), "file name str"="D:\\Data\\Ultrasound\\LSCO\\LSCO22__130814c\\5_Cooling_2nd_try\\September_2014\\091714\\55.06300K_500_2500_2.10000V_0.00000T_Sep17-2014__10-13-04_001_091714.bin", "mod time(min)"=58230133.06666667, "file format"=enum."binary", "power(V)"=2.1, "Magn Field(T) "=0.0}, {"temperature"=54.998, "temperature str"="54.99800", "file path"=path "D:/Data/Ultrasound/LSCO/LSCO22__130814c/5_Cooling_2nd_try/September_2014/091714/54.99800K_500_2500_2.10000V_0.00000T_Sep17-2014__10-14-23_001_091714.bin", "last mod"=timestamp(3493808063 s since 1904-01-01), "file name str"="D:\\Data\\Ultrasound\\LSCO\\LSCO22__130814c\\5_Cooling_2nd_try\\September_2014\\091714\\54.99800K_500_2500_2.10000V_0.00000T_Sep17-2014__10-14-23_001_091714.bin", "mod time(min)"=58230134.38333333, "file format"=enum."binary", "power(V)"=2.1, "Magn Field(T) "=0.0}, {"temperature"=54.938, "temperature str"="54.93800", "file path"=path "D:/Data/Ultrasound/LSCO/LSCO22__130814c/5_Cooling_2nd_try/September_2014/091714/54.93800K_500_2500_2.10000V_0.00000T_Sep17-2014__10-15-43_001_091714.bin", "last mod"=timestamp(3493808143 s since 1904-01-01), "file name str"="D:\\Data\\Ultrasound\\LSCO\\LSCO22__130814c\\5_Cooling_2nd_try\\September_2014\\091714\\54.93800K_500_2500_2.10000V_0.00000T_Sep17-2014__10-15-43_001_091714.bin", "mod time(min)"=58230135.71666667, "file format"=enum."binary", "power(V)"=2.1, "Magn Field(T) "=0.0}, {"temperature"=54.879, "temperature str"="54.87900", "file path"=path "D:/Data/Ultrasound/LSCO/LSCO22__130814c/5_Cooling_2nd_try/September_2014/091714/54.87900K_500_2500_2.10000V_0.00000T_Sep17-2014__10-17-02_001_091714.bin", "last mod"=timestamp(3493808222 s since 1904-01-01), "file name str"="D:\\Data\\Ultrasound\\LSCO\\LSCO22__130814c\\5_Cooling_2nd_try\\September_2014\\091714\\54.87900K_500_2500_2.10000V_0.00000T_Sep17-2014__10-17-02_001_091714.bin", "mod time(min)"=58230137.03333333, "file format"=enum."binary", "power(V)"=2.1, "Magn Field(T) "=0.0}, {"temperature"=54.816, "temperature str"="54.81600", "file path"=path "D:/Data/Ultrasound/LSCO/LSCO22__130814c/5_Cooling_2nd_try/September_2014/091714/54.81600K_500_2500_2.10000V_0.00000T_Sep17-2014__10-18-21_001_091714.bin", "last mod"=timestamp(3493808301 s since 1904-01-01), "file name str"="D:\\
